vi "Remove Element.vi"(8 "Error In":errorcluster, 10 "Element Tag":string, 11 "Display Manager In":refnum<class "Display Manager.lvclass">) -> (0 "Error Out":errorcluster, 3 "Display Manager Out":refnum<class "Display Manager.lvclass">)   [LabVIEW 2021, in "Display Manager.lvclass"]
uses:
  Display Manager.lvclass
  Display Element/Display Element.lvclass
  Display Manager.lvclass/Display Manager.ctl
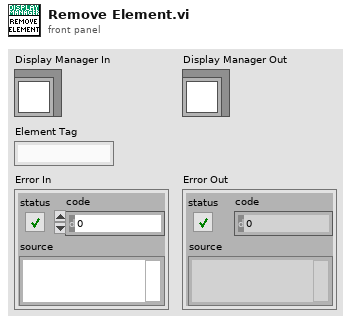
[diagram p1: front panel]
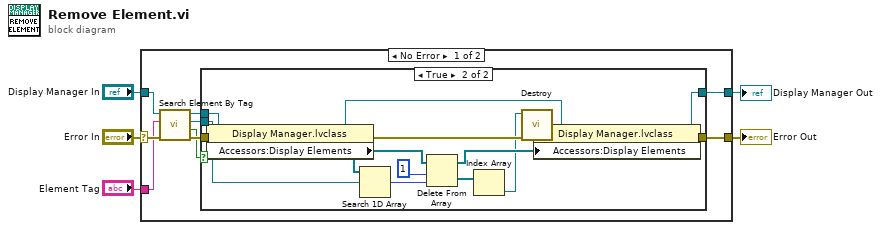
[diagram p0: block diagram]
diagram:
  n1 = case shown="No Error" "Error In" {
    selector: "Error In" -> [w12 w31]
    tunnel: "Display Manager In" -> [w11 w32]
    tunnel: [w13 w32] -> w3
    tunnel: [w14 w31] -> w2
    tunnel: "Element Tag" -> [w8 _]
    frame No Error {
      n2 = call "Search Element By Tag.vi"("Error In"=w12, "Element Tag"=w8, "Display Manager In"=w11) -> ("Error Out"=w10:errorcluster, "Found?"=w6:bool, "Display Element"=w7:refnum<class "Display Element.lvclass">, "Display Manager Out"=w9:refnum<class "Display Manager.lvclass">)  [unwired: 5 in]
      n3 = case shown="True" w6 {
        tunnel: [w15 w29] -> w14
        tunnel: [w16 w28] -> w13
        tunnel: w10 -> [w15 w23]
        tunnel: w9 -> [w16 w22]
        tunnel: w7 -> [_ w20]
        frame False {
        }
        frame True {
          n4 = property class="Display Manager.lvclass"(reference=w22, error in=w23) -> (reference out=w30:refnum<class "Display Manager.lvclass">, error out=w27:errorcluster, "Accessors:Display Elements"=w21:refnum<class "Display Element.lvclass">[])
          n5 = Search 1D Array(1D array=w21, element=w20) -> (index of element=w26:i32)  [unwired: 1 in]
          n6 = Delete From Array(array=w21, length=1, index=w26) -> (deleted portion=w18:refnum<class "Display Element.lvclass">[], array with subset deleted=w24:refnum<class "Display Element.lvclass">[])
          n7 = Index Array(array=w18) -> (element=w17:refnum<class "Display Element.lvclass">)  [unwired: 1 in]
          n8 = call-dynamic "Destroy.vi"("Error In"=w27, "Display Element In"=w17) -> ("Error Out"=w25:errorcluster)  [unwired: 9 in]
          n9 = property class="Display Manager.lvclass"(reference=w30, error in=w25, "Accessors:Display Elements"=w24) -> (reference out=w28:refnum<class "Display Manager.lvclass">, error out=w29:errorcluster)
        }
      }
    }
    frame Error {
    }
  }
  "Display Manager Out" <- w3
  "Error Out" <- w2
